vi "Sprinkler Controller.vi"() -> ()   [LabVIEW 2025]
uses:
  Controls/States.ctl
panel:
  in  "Zone Setup Array":cluster{"Zone Selector":string, "Timing":dbl}[](array[cluster])
  out "Controller Status":string
  out "Zone Indicators":T1
  in  "Water Pressure Sensor (%)":u32(slide) scale=0.0..100.0
  in  "Rain Sensor":bool
  in  "Run Selector":bool
  in  "Setup":bool
  in  "Start":bool
  in  "stop":bool
  # "Controls"
  # "Simulation Controls"
  # "Rain"
  # "No Rain"
  # "Continuous"
  # "Single"
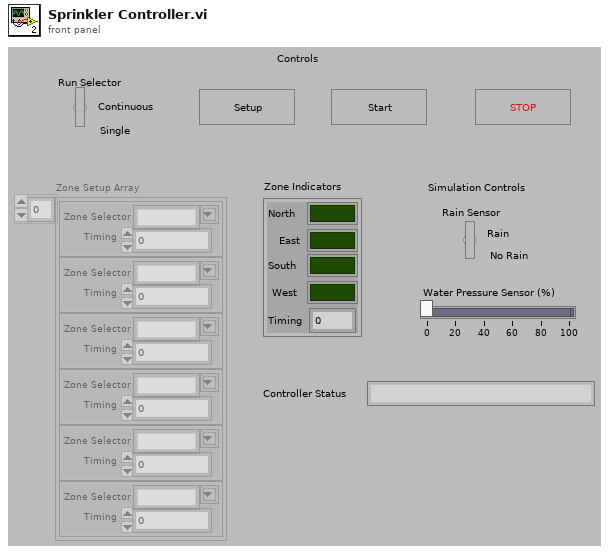
[diagram p1: front panel]
types:
  T1 = cluster{"North":bool, "East":bool, "South":bool, "West":bool, "Timing":u32}
  T2 = typedef "States.ctl" = enum16{"Initialization", "Wait For Start", "Setup", "Sprinkling Program", "North", "East", "South", "West", "Rain", "Low Water"}
  T3 = enum8{"Enabled", "Disabled", "Disabled and Grayed Out"}
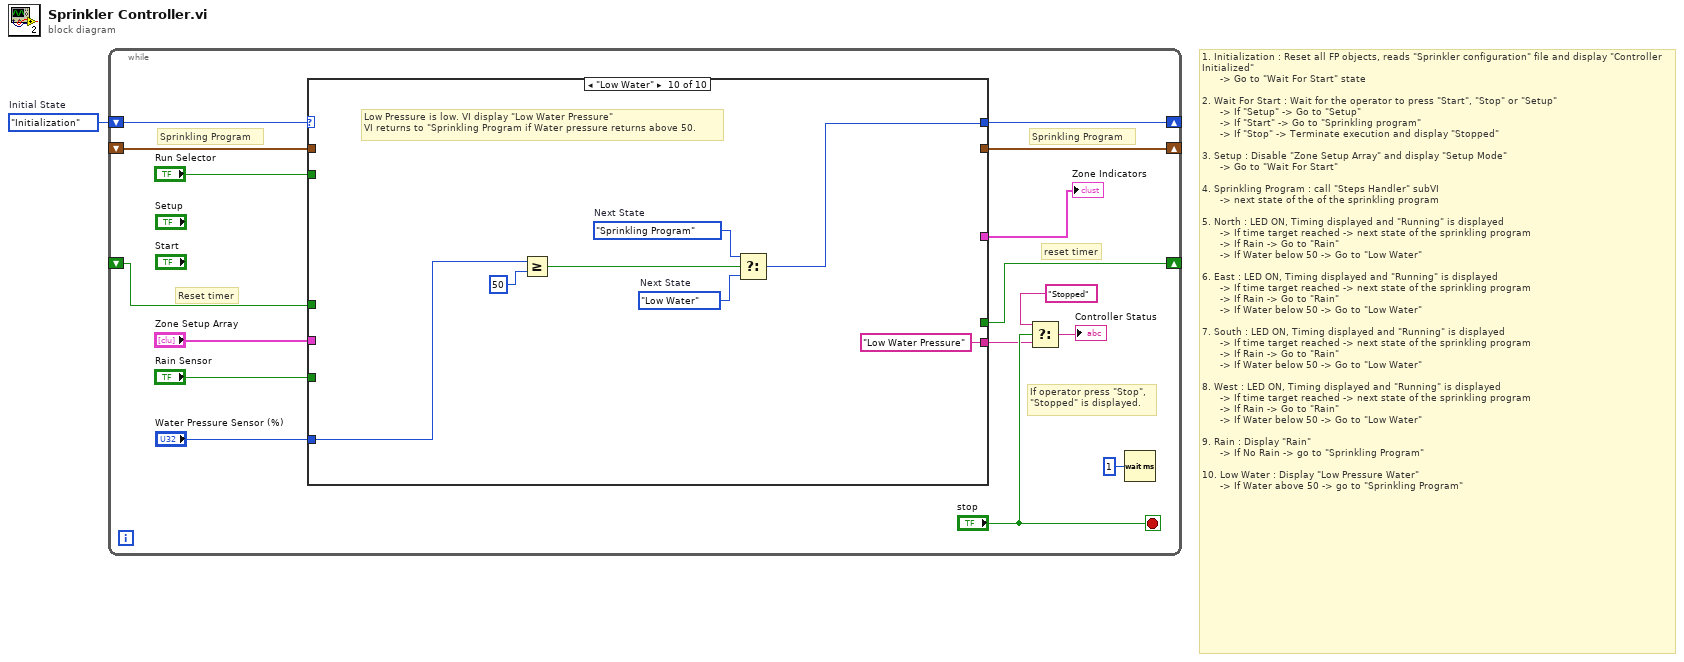
[diagram p0: block diagram]
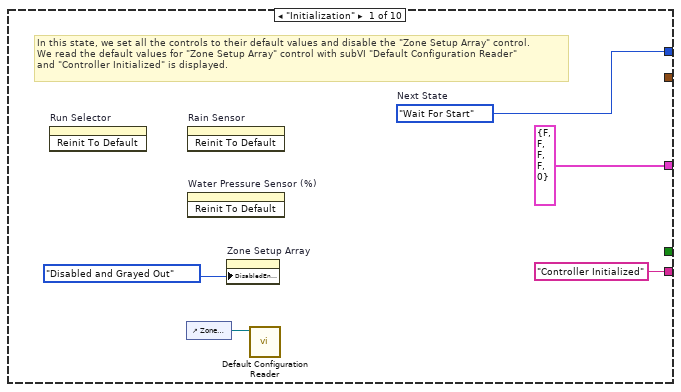
[diagram p2: hidden frame]
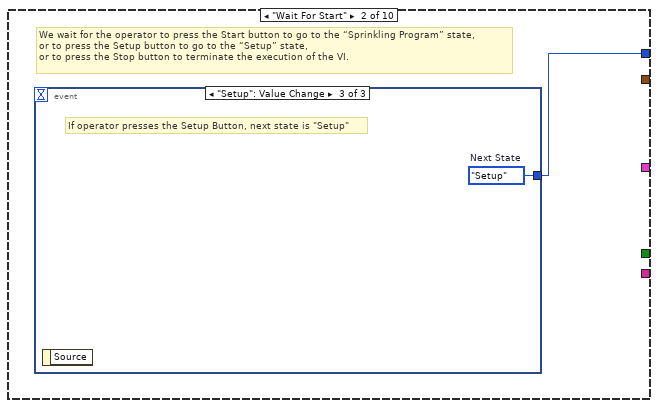
[diagram p3: hidden frame]
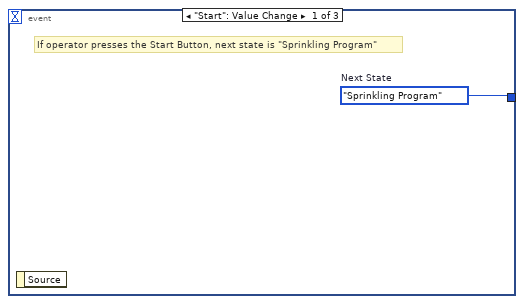
[diagram p4: hidden frame]
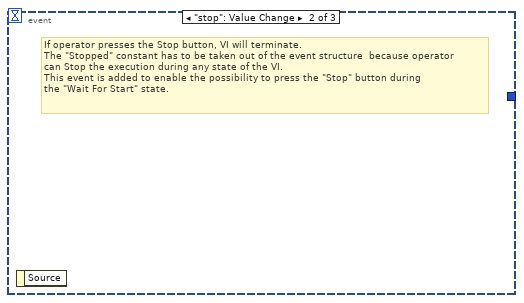
[diagram p5: hidden frame]
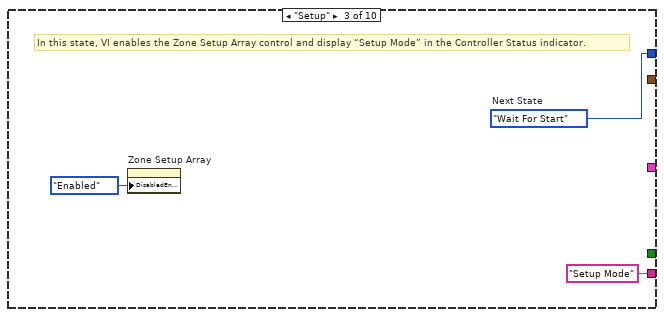
[diagram p6: hidden frame]
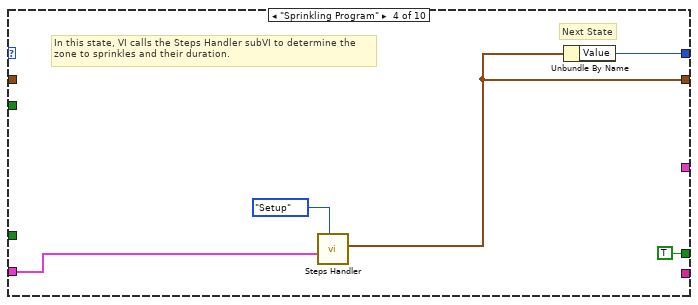
[diagram p7: hidden frame]
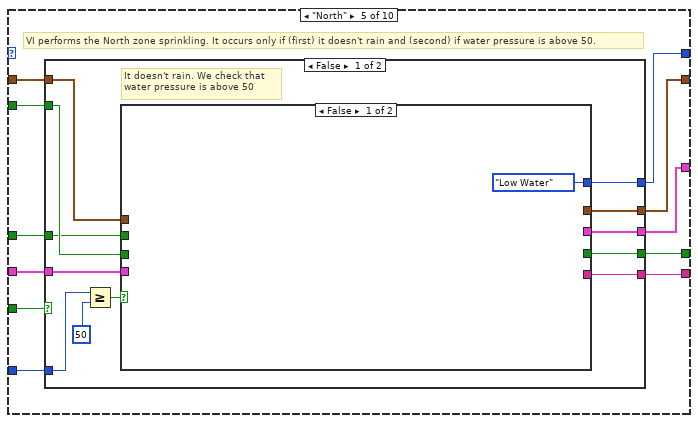
[diagram p8: hidden frame]
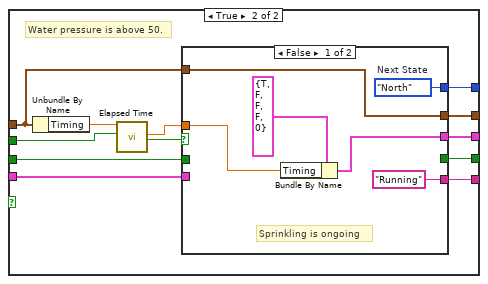
[diagram p9: hidden frame]
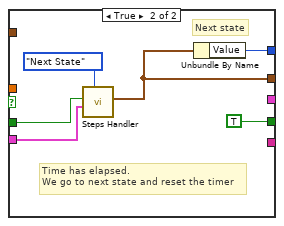
[diagram p10: hidden frame]
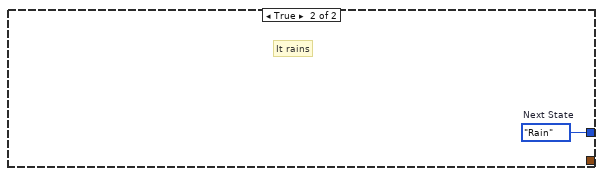
[diagram p11: hidden frame]
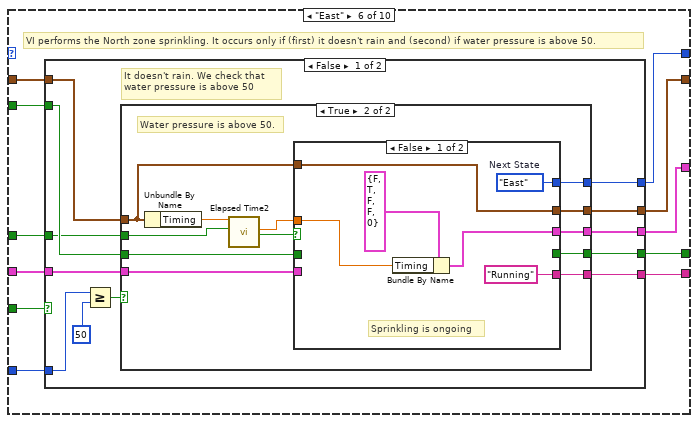
[diagram p12: hidden frame]
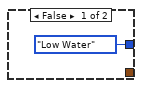
[diagram p13: hidden frame]
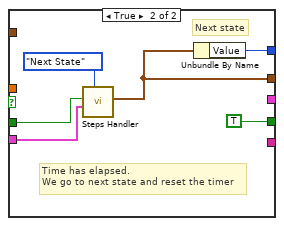
[diagram p14: hidden frame]
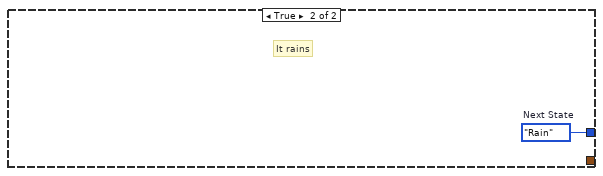
[diagram p15: hidden frame]
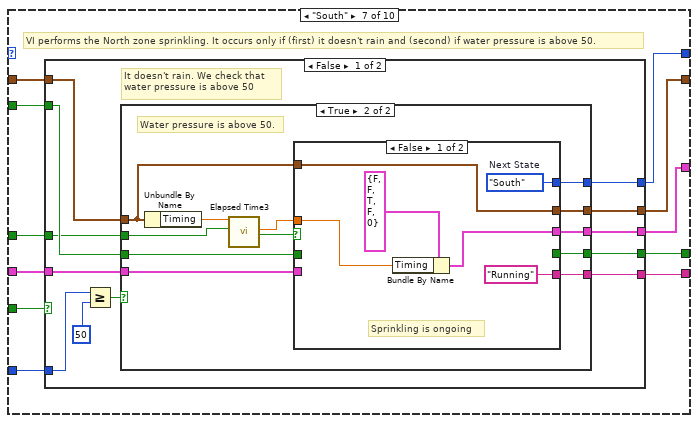
[diagram p16: hidden frame]
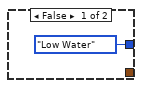
[diagram p17: hidden frame]
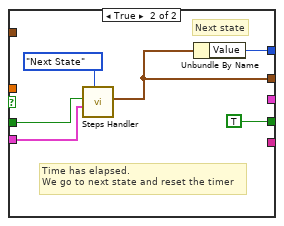
[diagram p18: hidden frame]
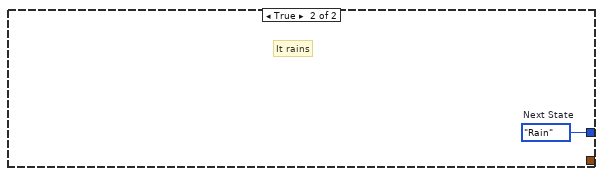
[diagram p19: hidden frame]
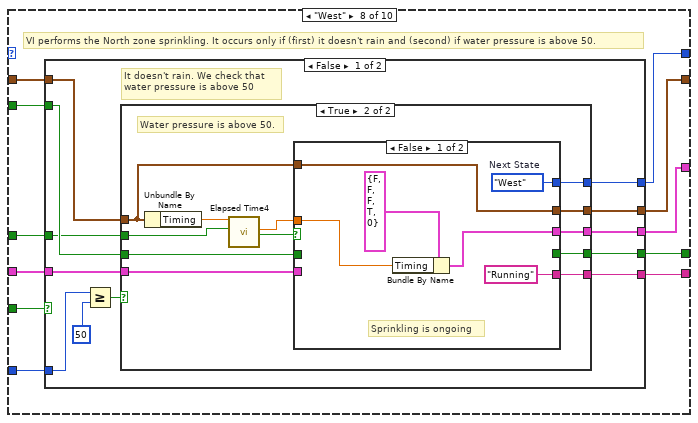
[diagram p20: hidden frame]
diagram:
  w1 = States."Initialization"  # Initial State
  # "1. Initialization : Reset all FP objects, reads \"Sprinkler configuration\" file and display \"Controller Initialized\"\n      -> Go to \"Wait For Start\" state\n\n2. Wait For Start : Wait for the operator to press \"Start\", \"Stop\" or \"Setup\"\n      -> If \"Setup\" -> Go to \"Setup\"\n      -> If \"Start\" -> Go to \"Sprinkling program\"\n      -> If \"Stop\" -> Terminate execution and display \"Stopped\"\n\n3. Setup : Disable \"Zone Setup Array\" and display \"Setup Mode\"\n      -> Go to \"Wait For Start\" \n\n4. Sprinkling Program : call \"Steps Handler\" subVI\n      -> next state of the of the sprinkling program\n\n5. North : LED ON, Timing displayed and \"Running\" is displayed\n      -> If time target reached -> next state of the sprinkling program\n      -> If Rain -> Go to \"Rain\"\n      -> If Water below 50 -> Go to \"Low Water\" \n\n6. East : LED ON, Timing displayed and \"Running\" is displayed\n      -> If time target reached -> next state of the sprinkling program\n      -> If Rain -> Go to \"Rain\"\n      -> If Water below 50 -> Go to \"Low Water\" \n\n7. South : LED ON, Timing displayed and \"Running\" is displayed\n      -> If time target reached -> next state of the sprinkling program\n      -> If Rain -> Go to \"Rain\"\n      -> If Water below 50 -> Go to \"Low Water\" \n\n8. West : LED ON, Timing displayed and \"Running\" is displayed\n      -> If time target reached -> next state of the sprinkling program\n      -> If Rain -> Go to \"Rain\"\n      -> If Water below 50 -> Go to \"Low Water\" \n\n9. Rain : Display \"Rain\"\n      -> If No Rain -> go to \"Sprinkling Program\"\n\n10. Low Water : Display \"Low Pressure Water\"\n      -> If Water above 50 -> go to \"Sprinkling Program\""
  n1 = while {
    shift-right: [w14] -> _
    shift-left: w1 -> [w17]
    shift-right: [w8] -> _
    shift-left: _ -> [w7]
    shift-right: [w3] -> _
    shift-left: _ -> [w2]
    stop <- "stop" stop-if-true
    # "reset timer"
    # "Reset timer"
    # "Sprinkling Program"
    # "Sprinkling Program"
    # "If operator press \"Stop\",\n\"Stopped\" is displayed."
    n2 = case shown="\"Low Water\"" w17 {
      tunnel: ["Controller Initialized" _ "Setup Mode" _ w34 w83 w132 w181 "Rain" "Low Water Pressure"] -> w12
      tunnel: [T1 {"North"=FALSE, "East"=FALSE, "South"=FALSE, "West"=FALSE, "Timing"=0} ("Zone Indicators") _ _ _ w35 w84 w133 w182 _ _] -> w15
      tunnel: [w18 w23 w27 w32 w44 w93 w142 w191 w231 w236] -> w14
      tunnel: "Zone Setup Array" -> [_ _ _ w30 w39 w88 w137 w186 _ _]
      tunnel: [_ _ _ w31 w38 w87 w136 w185 _ _] -> w8
      tunnel: w7 -> [_ _ _ _ w42 w91 w140 w189 _ _]
      tunnel: "Run Selector" -> [_ _ _ _ w40 w89 w138 w187 _ _]
      tunnel: "Rain Sensor" -> [_ _ _ _ w43 w92 w141 w190 w232 _]
      tunnel: "Water Pressure Sensor (%)" -> [_ _ _ _ w41 w90 w139 w188 _ w237]
      tunnel: [_ _ _ TRUE w37 w86 w135 w184 _ _] -> w3
      tunnel: w2 -> [_ _ _ _ w36 w85 w134 w183 _ _]
      frame "Initialization" {
        w18 = States."Wait For Start"  # Next State
        # "In this state, we set all the controls to their default values and disable the \"Zone Setup Array\" control.\nWe read the default values for \"Zone Setup Array\" control with subVI \"Default Configuration Reader\" \nand \"Controller Initialized\" is displayed."
        n3 = invoke on="Run Selector" class="Bool (strict)" method="Reinit To Default"() -> ()  [unwired: 3 in, 3 out]
        n4 = control-ref of="Zone Setup Array"() -> (w22:refnum<vi>)
        n5 = invoke on="Rain Sensor" class="Bool (strict)" method="Reinit To Default"() -> ()  [unwired: 3 in, 3 out]
        n6 = invoke on="Water Pressure Sensor (%)" class="Slide (strict)" method="Reinit To Default"() -> ()  [unwired: 3 in, 3 out]
        n7 = property on="Zone Setup Array" class="Arr (strict)"("DisabledEnum"=T3."Disabled and Grayed Out" ("Disabled")) -> ()  [unwired: 2 in, 2 out]
        n8 = call "Default Configuration Reader.vi"("Zone Setup Array ref"=w22) -> ()  [unwired: 11 in]
      }
      frame "Wait For Start" {
        # "We wait for the operator to press the Start button to go to the “Sprinkling Program” state, \nor to press the Setup button to go to the “Setup” state, \nor to press the Stop button to terminate the execution of the VI."
        n9 = event shown="[2] \"Setup\": Value Change" {
          selector: _ -> [_ _ _]
          dyn-events: _ -> [_ _ _]
          timeout: _ -> [_ _ _]
          tunnel: [w24 _ w25] -> w23
          event "Start": Value Change {
            w24 = States."Sprinkling Program"  # Next State
            # "If operator presses the Start Button, next state is \"Sprinkling Program\""
            n10 = event-data() -> ()  [unwired: 1 in, 1 out]
          }
          event "stop": Value Change {
            # "If operator presses the Stop button, VI will terminate.\nThe \"Stopped\" constant has to be taken out of the event structure  because operator\ncan Stop the execution during any state of the VI.\nThis event is added to enable the possibility to press the \"Stop\" button during \nthe \"Wait For Start\" state."
            n11 = event-data() -> ()  [unwired: 1 in, 1 out]
          }
          event "Setup": Value Change {
            w25 = States."Setup"  # Next State
            # "If operator presses the Setup Button, next state is \"Setup\""
            n12 = event-data() -> ()  [unwired: 1 in, 1 out]
          }
        }
      }
      frame "Setup" {
        w27 = States."Wait For Start"  # Next State
        # "In this state, VI enables the Zone Setup Array control and display “Setup Mode” in the Controller Status indicator."
        n13 = property on="Zone Setup Array" class="Arr (strict)"("DisabledEnum"=T3."Enabled" ("Disabled")) -> ()  [unwired: 2 in, 2 out]
      }
      frame "Sprinkling Program" {
        # "In this state, VI calls the Steps Handler subVI to determine the\nzone to sprinkles and their duration."
        # "Next State"
        n14 = call "Steps Handler.vi"("Operation"=enum16{"Setup", "Next State"}."Setup", "Zone Setup Array"=w30) -> ("Next State"=w31:cluster{"Value":T2, "Timing":dbl})  [unwired: 9 in]
        n15 = Unbundle By Name(w31) -> ("Value"=w32:T2)
      }
      frame "North" {
        # "VI performs the North zone sprinkling. It occurs only if (first) it doesn't rain and (second) if water pressure is above 50."
        n16 = case shown="False" w43 {
          tunnel: [w49 w82] -> w44
          tunnel: w42 -> [w53 _]
          tunnel: w41 -> [w56 _]
          tunnel: w40 -> [w52 _]
          tunnel: w39 -> [w51 _]
          tunnel: [w50 _] -> w38
          tunnel: [w48 _] -> w37
          tunnel: w36 -> [w47 _]
          tunnel: [w46 _] -> w35
          tunnel: [w45 _] -> w34
          frame False {
            # "It doesn't rain. We check that \nwater pressure is above 50"
            n17 = Greater Or Equal?(x=w56, y=u32 50) -> (x >= y?=w54:bool)
            n18 = case shown="False" w54 {
              tunnel: w53 -> [_ w61]
              tunnel: w52 -> [_ w67]
              tunnel: w51 -> [_ w66]
              tunnel: [_ w65] -> w50
              tunnel: [States."Low Water" ("Value") w64] -> w49
              tunnel: [_ w63] -> w48
              tunnel: w47 -> [_ w62]
              tunnel: [_ w59] -> w46
              tunnel: [_ w58] -> w45
              frame False {
              }
              frame True {
                # "Water pressure is above 50."
                n19 = Unbundle By Name(w61) -> ("Timing"=w69:dbl)
                n20 = call "Elapsed Time"("Time Target (s)"=w69, "Reset"=w62) -> ("Elapsed Time (s)"=w60:dbl, "Time has Elapsed"=w68:bool)  [unwired: 10 in, 6 out]
                n21 = case shown="False" w68 {
                  tunnel: w67 -> [_ w80]
                  tunnel: w66 -> [_ w79]
                  tunnel: [w74 w78] -> w65
                  tunnel: [w75 w77] -> w64
                  tunnel: [_ TRUE] -> w63
                  tunnel: w61 -> [w74 _]
                  tunnel: w60 -> [w70 _]
                  tunnel: [w72 _] -> w59
                  tunnel: ["Running" _] -> w58
                  frame False {
                    w75 = States."North"  # Next State
                    # "Sprinkling is ongoing"
                    n22 = Bundle By Name(cluster=T1 {"North"=TRUE, "East"=FALSE, "South"=FALSE, "West"=FALSE, "Timing"=0} ("Zone Indicators"), "Timing"=w70) -> (w72:T1)
                  }
                  frame True {
                    # "Next state"
                    # "Time has elapsed.\nWe go to next state and reset the timer"
                    n23 = call "Steps Handler.vi"("Operation"=enum16{"Setup", "Next State"}."Next State", "Zone Setup Array"=w79, "Run Selector"=w80) -> ("Next State"=w78:cluster{"Value":T2, "Timing":dbl})  [unwired: 8 in]
                    n24 = Unbundle By Name(w78) -> ("Value"=w77:T2)
                  }
                }
              }
            }
          }
          frame True {
            w82 = States."Rain"  # Next State
            # "It rains"
          }
        }
      }
      frame "East" {
        # "VI performs the North zone sprinkling. It occurs only if (first) it doesn't rain and (second) if water pressure is above 50."
        n25 = case shown="False" w92 {
          tunnel: [w98 w131] -> w93
          tunnel: w91 -> [w102 _]
          tunnel: w90 -> [w105 _]
          tunnel: w89 -> [w101 _]
          tunnel: w88 -> [w100 _]
          tunnel: [w99 _] -> w87
          tunnel: [w97 _] -> w86
          tunnel: w85 -> [w96 _]
          tunnel: [w95 _] -> w84
          tunnel: [w94 _] -> w83
          frame False {
            # "It doesn't rain. We check that \nwater pressure is above 50"
            n26 = Greater Or Equal?(x=w105, y=u32 50) -> (x >= y?=w103:bool)
            n27 = case shown="True" w103 {
              tunnel: w102 -> [_ w110]
              tunnel: w101 -> [_ w116]
              tunnel: w100 -> [_ w115]
              tunnel: [_ w114] -> w99
              tunnel: [States."Low Water" ("Value") w113] -> w98
              tunnel: [_ w112] -> w97
              tunnel: w96 -> [_ w111]
              tunnel: [_ w108] -> w95
              tunnel: [_ w107] -> w94
              frame False {
              }
              frame True {
                # "Water pressure is above 50."
                n28 = Unbundle By Name(w110) -> ("Timing"=w118:dbl)
                n29 = call "Elapsed Time2"("Time Target (s)"=w118, "Reset"=w111) -> ("Elapsed Time (s)"=w109:dbl, "Time has Elapsed"=w117:bool)  [unwired: 10 in, 6 out]
                n30 = case shown="False" w117 {
                  tunnel: w116 -> [_ w129]
                  tunnel: w115 -> [_ w128]
                  tunnel: [w123 w127] -> w114
                  tunnel: [w124 w126] -> w113
                  tunnel: [_ TRUE] -> w112
                  tunnel: w110 -> [w123 _]
                  tunnel: w109 -> [w119 _]
                  tunnel: [w121 _] -> w108
                  tunnel: ["Running" _] -> w107
                  frame False {
                    w124 = States."East"  # Next State
                    # "Sprinkling is ongoing"
                    n31 = Bundle By Name(cluster=T1 {"North"=FALSE, "East"=TRUE, "South"=FALSE, "West"=FALSE, "Timing"=0} ("Zone Indicators"), "Timing"=w119) -> (w121:T1)
                  }
                  frame True {
                    # "Next state"
                    # "Time has elapsed.\nWe go to next state and reset the timer"
                    n32 = call "Steps Handler.vi"("Operation"=enum16{"Setup", "Next State"}."Next State", "Zone Setup Array"=w128, "Run Selector"=w129) -> ("Next State"=w127:cluster{"Value":T2, "Timing":dbl})  [unwired: 8 in]
                    n33 = Unbundle By Name(w127) -> ("Value"=w126:T2)
                  }
                }
              }
            }
          }
          frame True {
            w131 = States."Rain"  # Next State
            # "It rains"
          }
        }
      }
      frame "South" {
        # "VI performs the North zone sprinkling. It occurs only if (first) it doesn't rain and (second) if water pressure is above 50."
        n34 = case shown="False" w141 {
          tunnel: [w147 w180] -> w142
          tunnel: w140 -> [w151 _]
          tunnel: w139 -> [w154 _]
          tunnel: w138 -> [w150 _]
          tunnel: w137 -> [w149 _]
          tunnel: [w148 _] -> w136
          tunnel: [w146 _] -> w135
          tunnel: w134 -> [w145 _]
          tunnel: [w144 _] -> w133
          tunnel: [w143 _] -> w132
          frame False {
            # "It doesn't rain. We check that \nwater pressure is above 50"
            n35 = Greater Or Equal?(x=w154, y=u32 50) -> (x >= y?=w152:bool)
            n36 = case shown="True" w152 {
              tunnel: w151 -> [_ w159]
              tunnel: w150 -> [_ w165]
              tunnel: w149 -> [_ w164]
              tunnel: [_ w163] -> w148
              tunnel: [States."Low Water" ("Value") w162] -> w147
              tunnel: [_ w161] -> w146
              tunnel: w145 -> [_ w160]
              tunnel: [_ w157] -> w144
              tunnel: [_ w156] -> w143
              frame False {
              }
              frame True {
                # "Water pressure is above 50."
                n37 = Unbundle By Name(w159) -> ("Timing"=w167:dbl)
                n38 = call "Elapsed Time3"("Time Target (s)"=w167, "Reset"=w160) -> ("Elapsed Time (s)"=w158:dbl, "Time has Elapsed"=w166:bool)  [unwired: 10 in, 6 out]
                n39 = case shown="False" w166 {
                  tunnel: w165 -> [_ w178]
                  tunnel: w164 -> [_ w177]
                  tunnel: [w172 w176] -> w163
                  tunnel: [w173 w175] -> w162
                  tunnel: [_ TRUE] -> w161
                  tunnel: w159 -> [w172 _]
                  tunnel: w158 -> [w168 _]
                  tunnel: [w170 _] -> w157
                  tunnel: ["Running" _] -> w156
                  frame False {
                    w173 = States."South"  # Next State
                    # "Sprinkling is ongoing"
                    n40 = Bundle By Name(cluster=T1 {"North"=FALSE, "East"=FALSE, "South"=TRUE, "West"=FALSE, "Timing"=0} ("Zone Indicators"), "Timing"=w168) -> (w170:T1)
                  }
                  frame True {
                    # "Next state"
                    # "Time has elapsed.\nWe go to next state and reset the timer"
                    n41 = call "Steps Handler.vi"("Operation"=enum16{"Setup", "Next State"}."Next State", "Zone Setup Array"=w177, "Run Selector"=w178) -> ("Next State"=w176:cluster{"Value":T2, "Timing":dbl})  [unwired: 8 in]
                    n42 = Unbundle By Name(w176) -> ("Value"=w175:T2)
                  }
                }
              }
            }
          }
          frame True {
            w180 = States."Rain"  # Next State
            # "It rains"
          }
        }
      }
      frame "West" {
        # "VI performs the North zone sprinkling. It occurs only if (first) it doesn't rain and (second) if water pressure is above 50."
        n43 = case shown="False" w190 {
          tunnel: [w196 w229] -> w191
          tunnel: w189 -> [w200 _]
          tunnel: w188 -> [w203 _]
          tunnel: w187 -> [w199 _]
          tunnel: w186 -> [w198 _]
          tunnel: [w197 _] -> w185
          tunnel: [w195 _] -> w184
          tunnel: w183 -> [w194 _]
          tunnel: [w193 _] -> w182
          tunnel: [w192 _] -> w181
          frame False {
            # "It doesn't rain. We check that \nwater pressure is above 50"
            n44 = Greater Or Equal?(x=w203, y=u32 50) -> (x >= y?=w201:bool)
            n45 = case shown="True" w201 {
              tunnel: w200 -> [_ w208]
              tunnel: w199 -> [_ w214]
              tunnel: w198 -> [_ w213]
              tunnel: [_ w212] -> w197
              tunnel: [States."Low Water" ("Value") w211] -> w196
              tunnel: [_ w210] -> w195
              tunnel: w194 -> [_ w209]
              tunnel: [_ w206] -> w193
              tunnel: [_ w205] -> w192
              frame False {
              }
              frame True {
                # "Water pressure is above 50."
                n46 = Unbundle By Name(w208) -> ("Timing"=w216:dbl)
                n47 = call "Elapsed Time4"("Time Target (s)"=w216, "Reset"=w209) -> ("Elapsed Time (s)"=w207:dbl, "Time has Elapsed"=w215:bool)  [unwired: 10 in, 6 out]
                n48 = case shown="False" w215 {
                  tunnel: w214 -> [_ w227]
                  tunnel: w213 -> [_ w226]
                  tunnel: [w221 w225] -> w212
                  tunnel: [w222 w224] -> w211
                  tunnel: [_ TRUE] -> w210
                  tunnel: w208 -> [w221 _]
                  tunnel: w207 -> [w217 _]
                  tunnel: [w219 _] -> w206
                  tunnel: ["Running" _] -> w205
                  frame False {
                    w222 = States."West"  # Next State
                    # "Sprinkling is ongoing"
                    n49 = Bundle By Name(cluster=T1 {"North"=FALSE, "East"=FALSE, "South"=FALSE, "West"=TRUE, "Timing"=0} ("Zone Indicators"), "Timing"=w217) -> (w219:T1)
                  }
                  frame True {
                    # "Next state"
                    # "Time has elapsed.\nWe go to next state and reset the timer"
                    n50 = call "Steps Handler.vi"("Operation"=enum16{"Setup", "Next State"}."Next State", "Zone Setup Array"=w226, "Run Selector"=w227) -> ("Next State"=w225:cluster{"Value":T2, "Timing":dbl})  [unwired: 8 in]
                    n51 = Unbundle By Name(w225) -> ("Value"=w224:T2)
                  }
                }
              }
            }
          }
          frame True {
            w229 = States."Rain"  # Next State
            # "It rains"
          }
        }
      }
      frame "Rain" {
        w234 = States."Sprinkling Program"  # Next State
        w233 = States."Rain"  # Next State
        # "It's rainning. VI display \"Rain\"\nVI returns to \"Sprinkling Program if it stops rainning."
        n52 = Select(t=w233, s=w232, f=w234) -> (s? t:f=w231:T2)
      }
      frame "Low Water" {
        w239 = States."Low Water"  # Next State
        w238 = States."Sprinkling Program"  # Next State
        # "Low Pressure is low. VI display \"Low Water Pressure\"\nVI returns to \"Sprinkling Program if Water pressure returns above 50."
        n53 = Greater Or Equal?(x=w237, y=u32 50) -> (x >= y?=w241:bool)
        n54 = Select(t=w238, s=w241, f=w239) -> (s? t:f=w236:T2)
      }
    }
    "Zone Indicators" <- w15
    n55 = Select(t="Stopped", s="stop", f=w12) -> (s? t:f=→"Controller Status":string)
    n56 = Wait (ms)(milliseconds to wait=u32 1) -> ()  [unwired: 1 out]
  }
